vi "GetUTC.vi"() -> (0 "UTC_fractional":dbl format="%.6g", 1 "Day":dbl, 2 "Month":dbl, 3 "Year":dbl, 4 "DST?":bool, 5 "UTC_seconds":dbl format="%<%H:%M:%S%1u>t", 6 "LST+_seconds":dbl format="%<%H:%M:%S%1u>t", 7 "LST_fractional":dbl format="%.6f", 8 "Julian Day":dbl format="%.12f")   [LabVIEW 2011]
panel:
  out "UTC_offset":i32
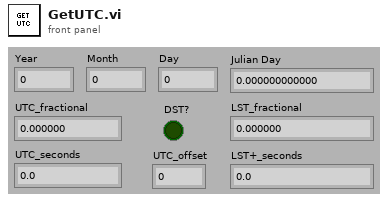
[diagram p1: front panel]
types:
  T1 = typedef "LVDateTimeRec.ctl" = cluster{"fractional second":dbl, "second":i32, "minute":i32, "hour":i32, "day of month":i32, "month":i32, "year":i32, "day of week":i32, "day of year":i32, "DST":i32}
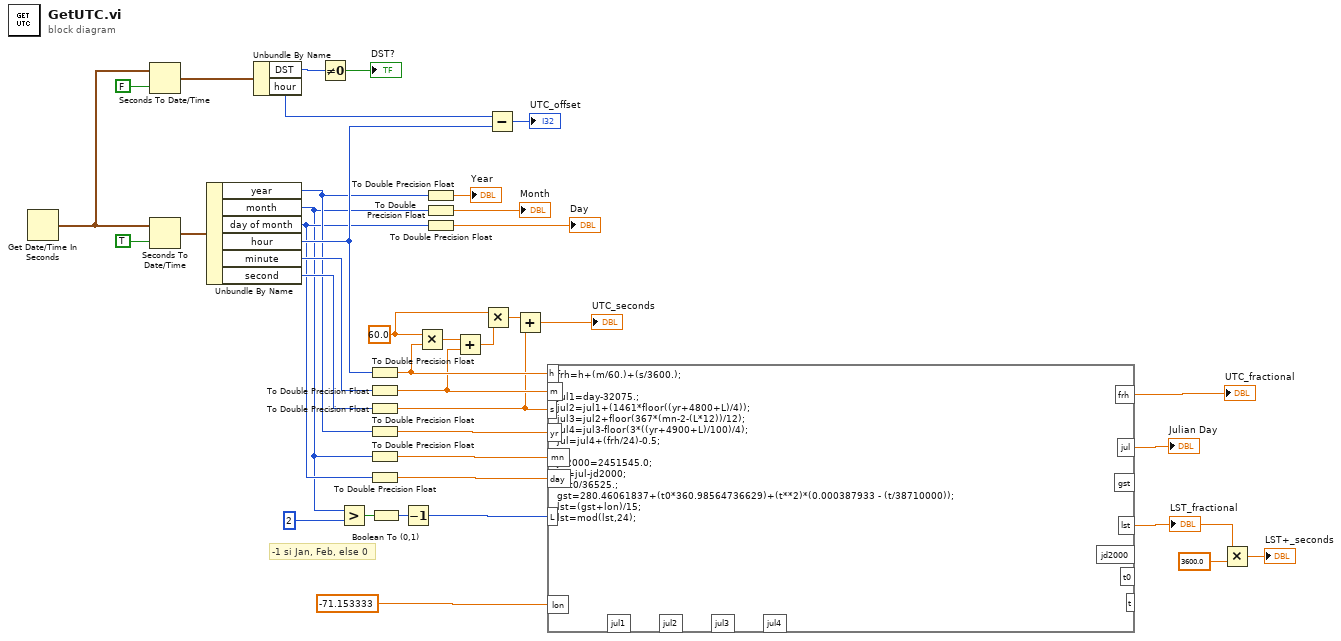
[diagram p0: block diagram]
diagram:
  w7 = 60.0
  # "-1 si Jan, Feb, else 0"
  n1 = Get Date/Time In Seconds() -> (seconds since 1Jan1904=w31:timestamp)
  n2 = Seconds To Date/Time(time stamp (now)=w31, to UTC (F)=FALSE) -> (date time rec=w30:T1)
  n3 = Seconds To Date/Time(time stamp (now)=w31, to UTC (F)=TRUE) -> (date time rec=w38:T1)
  n4 = Unbundle By Name(w38) -> ("year"=w23:i32, "month"=w17:i32, "day of month"=w22:i32, "hour"=w27:i32, "minute"=w37:i32, "second"=w36:i32)
  n5 = Unbundle By Name(w30) -> ("DST"=w29:i32, "hour"=w26:i32)
  n6 = Not Equal To 0?(x=w29) -> (x != 0?=→"DST?":bool)
  n7 = Greater?(x=w17, y=2) -> (0:w15:bool)
  n8 = To Double Precision Float(number=w27) -> (double precision float=w8:dbl)
  n9 = To Double Precision Float(number=w37) -> (double precision float=w5:dbl)
  n10 = To Double Precision Float(number=w36) -> (double precision float=w2:dbl)
  n11 = To Double Precision Float(number=w23) -> (double precision float=w21:dbl)
  n12 = To Double Precision Float(number=w17) -> (double precision float=w20:dbl)
  n13 = To Double Precision Float(number=w22) -> (double precision float=w19:dbl)
  n14 = Boolean To (0,1)(Boolean=w15) -> (0, 1=w14:i16)
  n15 = Decrement(x=w14) -> (x-1=w13:i16)
  n16 = Multiply(x=w7, y=w8) -> (x*y=w6:dbl)
  n17 = To Double Precision Float(number=w23) -> (double precision float=→"Year":dbl)
  n18 = To Double Precision Float(number=w17) -> (double precision float=→"Month":dbl)
  n19 = To Double Precision Float(number=w22) -> (double precision float=→"Day":dbl)
  n20 = Add(x=w6, y=w5) -> (x+y=w4:dbl)
  n21 = Multiply(x=w7, y=w4) -> (x*y=w3:dbl)
  n22 = Subtract(x=w26, y=w27) -> (x-y=→"UTC_offset":i32)
  n23 = Add(x=w3, y=w2) -> (x+y=→"UTC_seconds":dbl)
  n24 = formula code="frh=h+(m/60.)+(s/3600.);\n\njul1=day-32075.;\njul2=jul1+(1461*floor((yr+4800+L)/4));\njul3=jul2+floor(367*(mn-2-(L*12))/12);\njul4=jul3-floor(3*((yr+4900+L)/100)/4);\njul=jul4+(frh/24)-0.5;\n\njd2000=2451545.0;\nt0=jul-jd2000;\nt=t0/36525.;\ngst=280.46061837+(t0*360.98564736629)+(t**2)*(0.000387933 - (t/38710000));\nlst=(gst+lon)/15;\nlst=mod(lst,24);"("h"=w8, "m"=w5, "s"=w2, "lon"=-71.153333, "yr"=w21, "mn"=w20, "day"=w19, "L"=w13) -> ("frh"=→"UTC_fractional":dbl, "jul"=→"Julian Day":dbl, "lst"=w12:dbl)  [unwired: 8 out]
  "LST_fractional" <- w12
  n25 = Multiply(x=w12, y=3600.0) -> (x*y=→"LST+_seconds":dbl)
